vi "Dual Source Validation Utility.vi"(0 "Method File:":path=path "C:/Users/Public/Molana/Instrument/Project/MS Methods/MethodFile.xml") -> ()   [LabVIEW 2012]
uses:
  _XML Source Type.ctl
  _Source Parameter.ctl
  _Source Properties.ctl
  <vilib>/Utility/config.llb/Read Key (String).vi
  Configuration/_Global Configuration.vi
  <vilib>/xml/Close Reference(Node).vi
  <vilib>/xml/NI_XML.lvlib
  <resource>/objmgr/DOMUserDefRef.rc
  <vilib>/Utility/config.llb/NI_LVConfig.lvlib
panel:
  out "xml 2":string
  out "SourceProperties":T1[](array[typedef]) {"Source Type" items=["APCI 1", "APCI 2", "ESI 1", "ESI 2"]}
  out "Result":string="Press Load Method button to start"
  in  "Load":bool
  in  "Cancel":bool
  in  "Save As":bool
  in  "Save":bool
  out "xml":string
  in  "Current Expt":u16(ring) items=["0", "1"]
  in  "Tab":T3(tab)=enum."Experiments"
  out "Method-Level Parameter":string[][](table)
  out "Experiment List":string[][](table)
  out "Expt Comment":string
  out "Expt-Level Parameter":string[][](table)
  out "Source Type":T2 items=["APCI 1", "APCI 2", "ESI 1", "ESI 2"]
  out "Expt-Level Source Parameters":T4
  out "Mass Ranges":string[][](table)
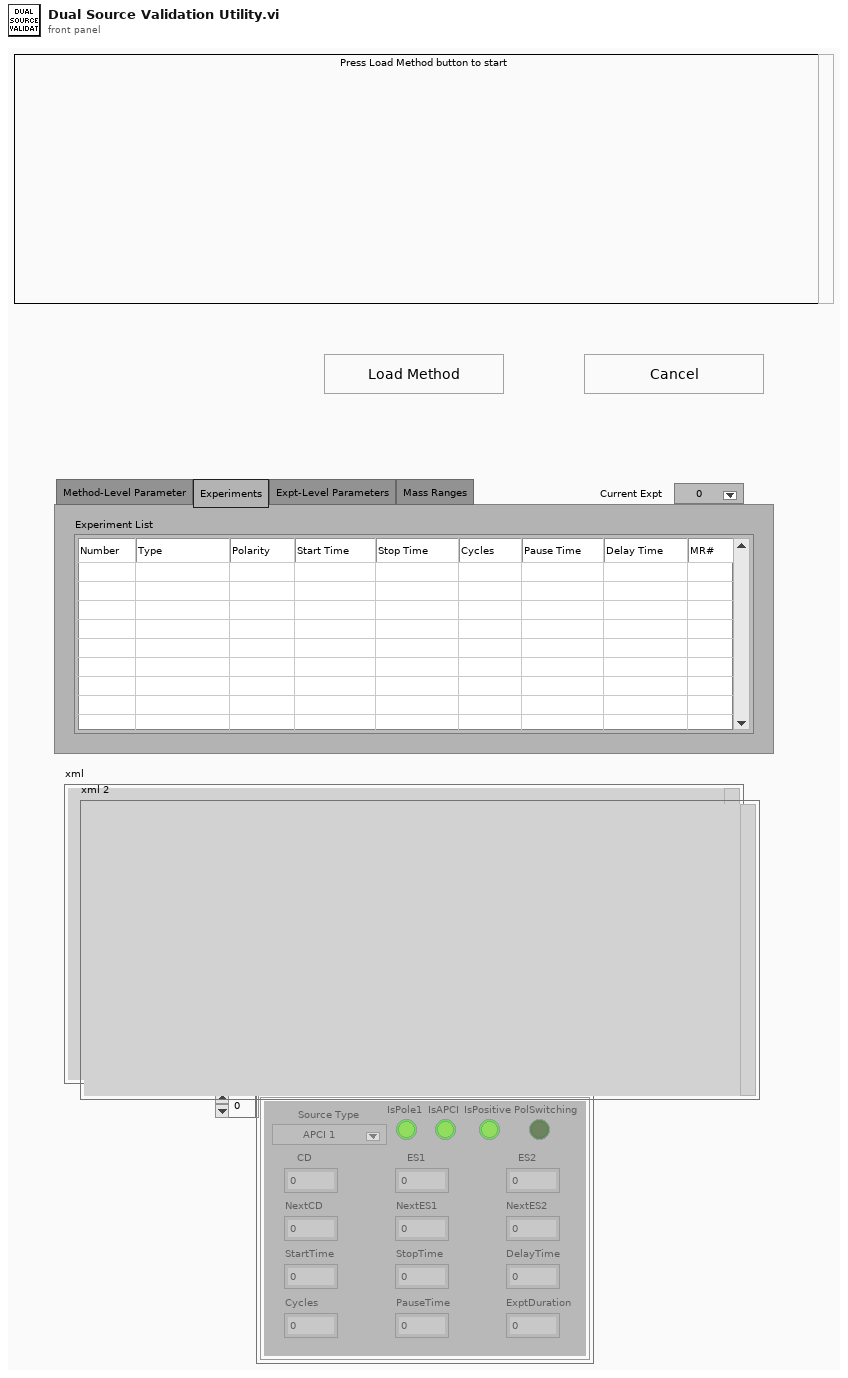
[diagram p1: front panel]
types:
  T1 = typedef "_Source Properties.ctl" = cluster{"Source Type":T2, "IsPole1":bool, "IsAPCI":bool, "IsPositive":bool, "CD":dbl, "ES1":dbl, "ES2":dbl, "NextCD":dbl, "NextES1":dbl, "NextES2":dbl, "PolSwitching":bool, "StartTime":dbl, "StopTime":dbl, "DelayTime":dbl, "Cycles":i32, "PauseTime":dbl, "ExptDuration":dbl}
  T2 = typedef "_XML Source Type.ctl" = u16
  T3 = enum32{"Method-Level Parameter", "Experiments", "Expt-Level Parameters", "Mass Ranges"}
  T4 = typedef "_Source Parameter.ctl" = cluster{"Corona Discharge: ":dbl, "ElectroSpray V1: ":dbl, "ElectroSpray V2: ":dbl}
  T5 = enum32{"existing file", "new file", "new or existing file", "existing dir", "new dir", "new or existing dir", "existing file (use LLBs)", "new file (use LLBs)", "new or existing file (use LLBs)", "new or existing file or directory (use LLBs)"}
  T6 = typedef "NI_LVConfig.lvlib/Config Data RefNum.ctl" = refnum<k1>
  T7 = typedef "_RT Instrument 2.ctl" = cluster{"Table":T8[], "Instrument":string[]}
  T8 = typedef "_RT Configuration 2.ctl" = cluster{"Name":string, "Ch#":u8, "Min":dbl, "Max":dbl, "Def+":dbl, "Def-":dbl, "Offset":dbl, "Slope":dbl, "Type":u8, "Description":string, "SettleT":dbl}
  T9 = typedef "_Mass Range Parameters.ctl" = cluster{"Name":string, "Ch#":u8, "StartV":dbl, "StopV":dbl, "StepV":dbl, "Index":u8}
  T10 = cluster{"ExptLevelParameters":string[][], "MassRanges":string[][], " MRParameters":T9[][]}
  T11 = cluster{"ExptLevelParameters":string[][], "MassRanges":string[][], " MRParameters":T9[][]}[]
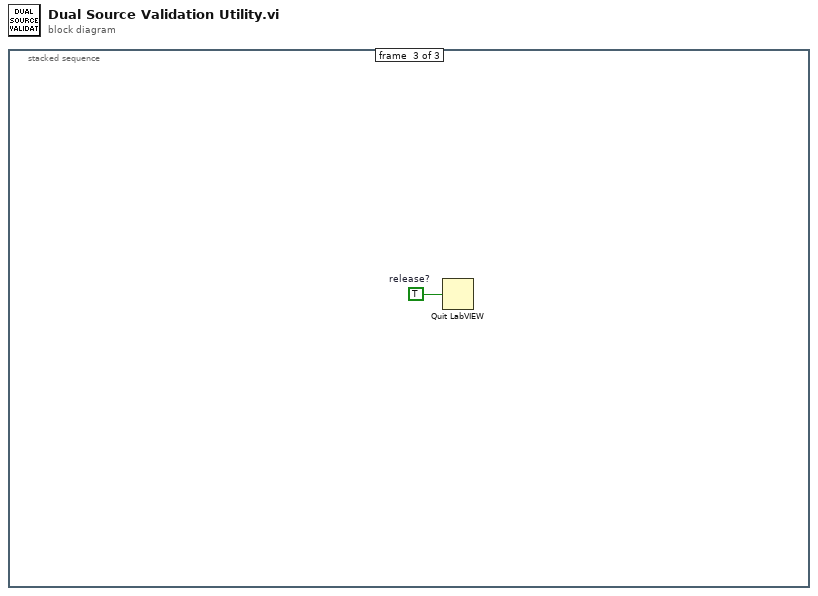
[diagram p0: block diagram]
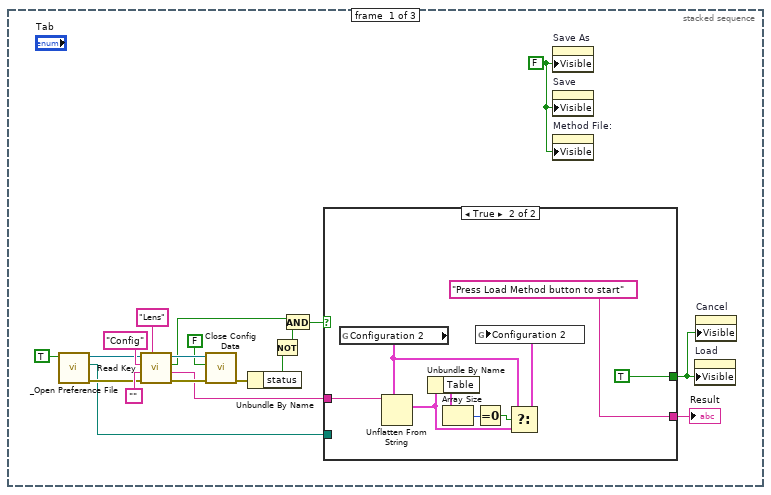
[diagram p2: hidden frame]
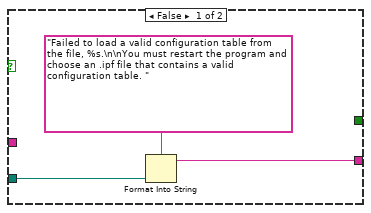
[diagram p3: hidden frame]
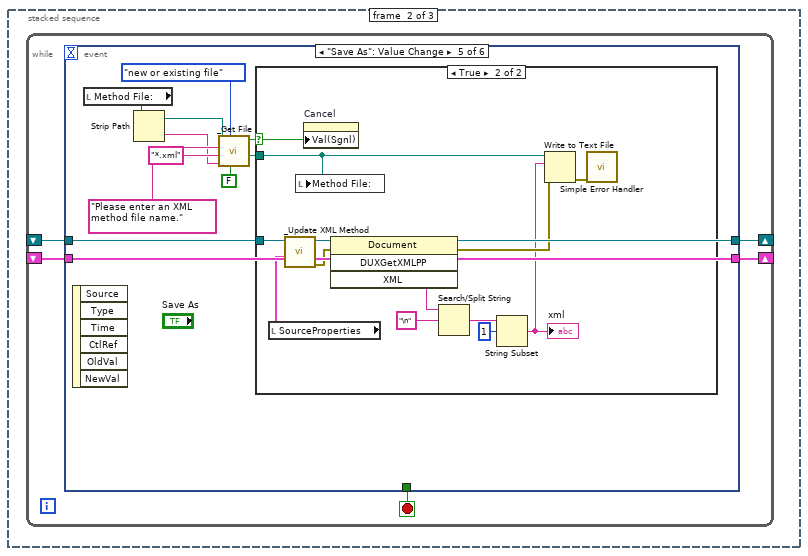
[diagram p4: hidden frame]
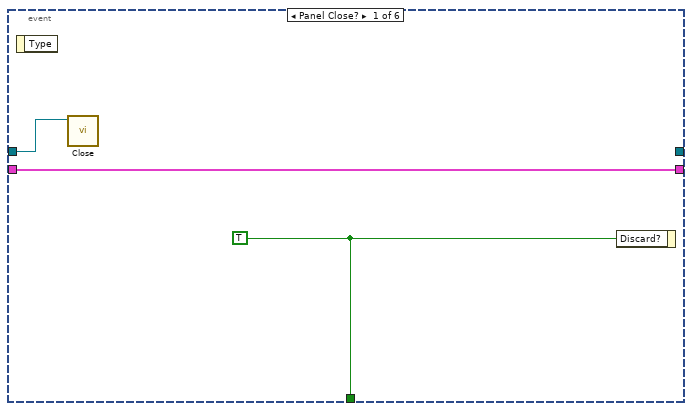
[diagram p5: hidden frame]
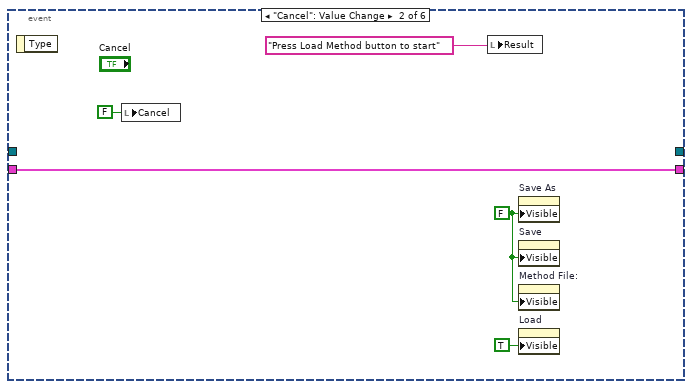
[diagram p6: hidden frame]
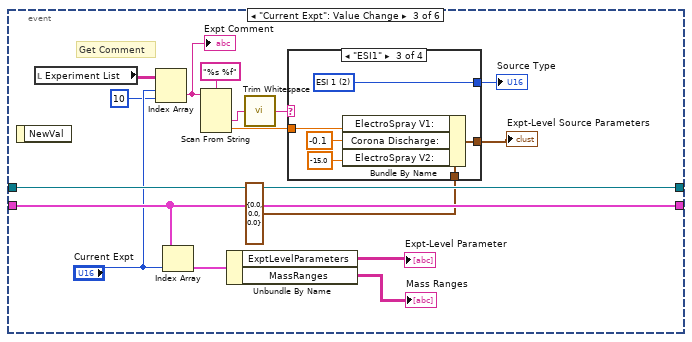
[diagram p7: hidden frame]
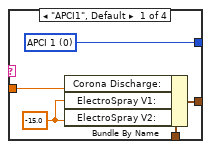
[diagram p8: hidden frame]
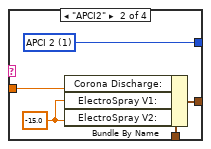
[diagram p9: hidden frame]
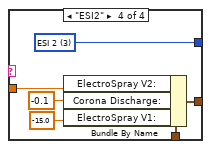
[diagram p10: hidden frame]
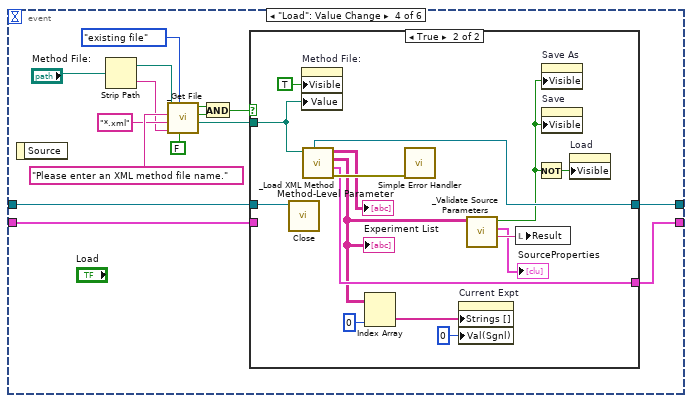
[diagram p11: hidden frame]
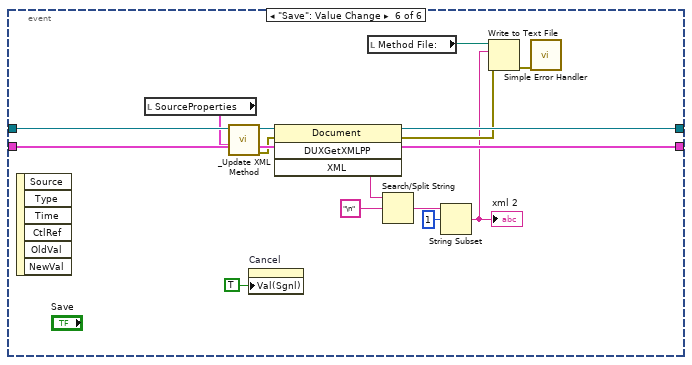
[diagram p14: hidden frame]
diagram:
  n1 = stacked-sequence {
    frame #0 {
      w7 = FALSE ("Visible")
      n2 = call "_Open Preference File.vi"("Use Designated"=TRUE) -> ("error"=w15:errorcluster, "ipf path"=w10:path, "refnum"=w16:T6)  [unwired: 4 out]
      n3 = call-poly <vilib>:"Read Key.vi"("section"="Lens", "error in (no error)"=w15, "default value"="", "key"="Config" ("section"), "refnum"=w16) -> ("error out"=w12:errorcluster, "value"=w11:string, "found?"=w3:bool, "refnum out"=w14:T6)  [unwired: 1 in, 2 out]
      n4 = call <vilib>:"Close Config Data.vi"("error in (no error)"=w12, "write file if changed (T)"=FALSE, "refnum"=w14) -> ("error out"=w6:errorcluster)  [unwired: 8 out]
      n5 = Unbundle By Name(w6) -> ("status"=w5:bool)
      n6 = Not(x=w5) -> (.not. x?=w4:bool)
      n7 = And(x=w3, y=w4) -> (x .and. y?=w2:bool)
      n8 = case shown="True" w2 {
        tunnel: w11 -> [_ w30]
        tunnel: w10 -> [w22 _]
        tunnel: [w20 "Press Load Method button to start" ("format string")] -> w8
        tunnel: [_ TRUE ("Visible")] -> w1
        frame False {
          n9 = Format Into String(format string="Failed to load a valid configuration table from the file, %s.\n\nYou must restart the program and choose an .ipf file that contains a valid configuration table. ", w22) -> (resulting string=w20:string)  [unwired: 2 in, 1 out]
        }
        frame True {
          n10 = global read "_Global Configuration.vi" "Configuration 2"() -> (w26:T7)
          n11 = Unflatten From String(type=w26, binary string=w30) -> (value=w25:T7)  [unwired: 1 in, 4 out]
          n12 = Unbundle By Name(w25) -> ("Table"=w29:T8[])
          n13 = Array Size(array=w29) -> (size(s)=w28:i32)
          n14 = Equal To 0?(x=w28) -> (x = 0?=w27:bool)
          n15 = Select(t=w26, s=w27, f=w25) -> (s? t:f=w24:T7)
          n16 = global write "_Global Configuration.vi" "Configuration 2"(w24) -> ()
        }
      }
      "Result" <- w8
      n17 = property on="Save As" class="Bool"("Visible"=w7) -> ()  [unwired: 2 in, 2 out]
      n18 = property on="Save" class="Bool"("Visible"=w7) -> ()  [unwired: 2 in, 2 out]
      n19 = property on="Method File:" class="Path"("Visible"=w7) -> ()  [unwired: 2 in, 2 out]
      n20 = property on="Load" class="Bool"("Visible"=w1) -> ()  [unwired: 2 in, 2 out]
      n21 = property on="Cancel" class="Bool (strict)"("Visible"=w1) -> ()  [unwired: 2 in, 2 out]
    }
    frame #1 {
      n22 = while {
        shift-right: [w34] -> _
        shift-left: _ -> [w35]
        shift-right: [w32] -> _
        shift-left: _ -> [w33]
        stop <- w36 stop-if-true
        n23 = event shown="[4] \"Save As\": Value Change" {
          selector: _ -> [_ _ _ _ _ _]
          dyn-events: _ -> [_ _ _ _ _ _]
          timeout: _ -> [_ _ _ _ _ _]
          tunnel: [w39 _ _ _ _ _] -> w36
          tunnel: w35 -> [w38 w44 w60 w88 w115 w151]
          tunnel: [w38 w44 w60 w89 w115 w151] -> w34
          tunnel: w33 -> [w37 _ w56 w87 w116 w152]
          tunnel: [_ _ w56 w86 w116 w152] -> w32
          event Panel Close? {
            w39 = TRUE ("Discard?")
            n24 = event-data() -> ()  [unwired: 2 out]
            n25 = call-poly <vilib>:"Close.vi"("node"=w37) -> ()  [unwired: 8 in, 1 out]
            n26 = event-data("Discard?"=w39) -> ()  [unwired: 1 in, 1 out]
          }
          event "Cancel": Value Change {
            w42 = FALSE ("Visible")
            n27 = event-data() -> ()  [unwired: 2 out]
            n28 = local write "Cancel"(FALSE ("Cancel")) -> ()
            n29 = local write "Result"("Press Load Method button to start" ("Result")) -> ()
            n30 = property on="Save As" class="Bool"("Visible"=w42) -> ()  [unwired: 2 in, 2 out]
            n31 = property on="Save" class="Bool"("Visible"=w42) -> ()  [unwired: 2 in, 2 out]
            n32 = property on="Method File:" class="Path"("Visible"=w42) -> ()  [unwired: 2 in, 2 out]
            n33 = property on="Load" class="Bool"("Visible"=TRUE) -> ()  [unwired: 2 in, 2 out]
          }
          event "Current Expt": Value Change {
            # "Get Comment"
            n34 = event-data() -> ()  [unwired: 2 out]
            n35 = local read "Experiment List"() -> (w55:string[][])
            n36 = Index Array(array=w55, index (row)="Current Expt", index (col)=10 ("disabled index (col)")) -> (element=w51:string)
            "Expt Comment" <- w51
            n37 = Index Array(array=w60, index="Current Expt") -> (element=w59:T10)
            n38 = Scan From String(format string="%s %f", input string=w51) -> (output 1=w50:string, output 2=w46:dbl)  [unwired: 4 in, 3 out]
            n39 = Unbundle By Name(w59) -> ("ExptLevelParameters"=→"Expt-Level Parameter":string[][], "MassRanges"=→"Mass Ranges":string[][])
            n40 = call <vilib>:"Trim Whitespace.vi"("string"=w50) -> ("trimmed string"=w49:string)  [unwired: 1 in]
            n41 = case shown="\"ESI1\"" w49 {
              tunnel: [w65 w70 w76 w82] -> w48
              tunnel: T4 {"Corona Discharge: "=0.0, "ElectroSpray V1: "=0.0, "ElectroSpray V2: "=0.0} ("Method-Level Source Parameters") -> [w64 w68 w73 w81]
              tunnel: w46 -> [w63 w67 w72 w80]
              tunnel: [w61 w66 w71 w77] -> w45
              frame "APCI1", Default {
                w62 = -15.0 ("ElectroSpray V2:")
                w65 = T2 0 items=["APCI 1", "APCI 2", "ESI 1", "ESI 2"] ("Source Type")
                n42 = Bundle By Name(cluster=w64, "Corona Discharge:"=w63, "ElectroSpray V1:"=w62, "ElectroSpray V2:"=w62) -> (w61:T4)
              }
              frame "APCI2" {
                w69 = -15.0 ("ElectroSpray V2:")
                w70 = T2 1 items=["APCI 1", "APCI 2", "ESI 1", "ESI 2"] ("Source Type")
                n43 = Bundle By Name(cluster=w68, "Corona Discharge:"=w67, "ElectroSpray V1:"=w69, "ElectroSpray V2:"=w69) -> (w66:T4)
              }
              frame "ESI1" {
                w76 = T2 2 items=["APCI 1", "APCI 2", "ESI 1", "ESI 2"] ("Source Type")
                n44 = Bundle By Name(cluster=w73, "ElectroSpray V1:"=w72, "Corona Discharge:"=-0.1, "ElectroSpray V2:"=-15.0) -> (w71:T4)
              }
              frame "ESI2" {
                w82 = T2 3 items=["APCI 1", "APCI 2", "ESI 1", "ESI 2"] ("Source Type")
                n45 = Bundle By Name(cluster=w81, "ElectroSpray V2:"=w80, "Corona Discharge:"=-0.1, "ElectroSpray V1:"=-15.0 ("ElectroSpray V2:")) -> (w77:T4)
              }
            }
            "Source Type" <- w48
            "Expt-Level Source Parameters" <- w45
          }
          event "Load": Value Change {
            n46 = event-data() -> ()  [unwired: 2 out]
            n47 = Strip Path(path="Method File:") -> (stripped path=w84:path, name=w83:string)
            n48 = call "_Get File.vi"("For Write (T)"=FALSE, "select mode (new or existing)"=T5."existing file", "default name"=w83, "extension (isd)"="*.xml", "prompt"="Please enter an XML method file name.", "Start Path"=w84) -> ("Seleted File"=w90:path, "Exists"=w92:bool, "Succeeded"=w93:bool)  [unwired: 1 in]
            n49 = And(x=w93, y=w92) -> (x .and. y?=w91:bool)
            n50 = case shown="True" w91 {
              tunnel: w90 -> [_ w106]
              tunnel: [w99 w112] -> w89
              tunnel: w88 -> [w99 _]
              tunnel: w87 -> [w98 w107]
              tunnel: [w98 w108] -> w86
              frame False {
              }
              frame True {
                n51 = call-poly <vilib>:"Close.vi"("node"=w107) -> ()  [unwired: 8 in, 1 out]
                n52 = property on="Method File:" class="Path"("Visible"=TRUE, "Value"=w106) -> ()  [unwired: 2 in, 2 out]
                n53 = call "_Load XML Method.vi"("Path"=w106) -> ("error out"=w114:errorcluster, "ExptParamAndMR"=w112:T11, "Experiment List"=w103:string[][], "MethodLevelParameters"=→"Method-Level Parameter":string[][], "DOM document"=w108:refnum<k20>)  [unwired: 3 in]
                "Experiment List" <- w103
                n54 = Index Array(array=w103, index (col)=0 ("disabled index (col)")) -> (element=w110:string[])  [unwired: 1 in]
                n55 = call <vilib>:"Simple Error Handler.vi"("error in (no error)"=w114) -> ()  [unwired: 4 in, 5 out]
                n56 = property on="Current Expt" class="Ring (strict)"("Strings []"=w110, "Val(Sgnl)"=u16 0 ("Value (Signaling)")) -> ()  [unwired: 2 in, 2 out]
                n57 = call "_Validate Source Parameters.vi"("Expts"=w103) -> ("Error"=w102:string, "SourceProperties"=→"SourceProperties":T1[], "Valid"=w101:bool)  [unwired: 8 in]
                n58 = local write "Result"(w102) -> ()
                n59 = Not(x=w101) -> (.not. x?=w104:bool)
                n60 = property on="Save As" class="Bool"("Visible"=w101) -> ()  [unwired: 2 in, 2 out]
                n61 = property on="Save" class="Bool"("Visible"=w101) -> ()  [unwired: 2 in, 2 out]
                n62 = property on="Load" class="Bool"("Visible"=w104) -> ()  [unwired: 2 in, 2 out]
              }
            }
          }
          event "Save As": Value Change {
            n63 = event-data() -> ()  [unwired: 7 out]
            n64 = local read "Method File:"() -> (w121:path)
            n65 = Strip Path(path=w121) -> (stripped path=w120:path, name=w119:string)
            n66 = call "_Get File.vi"("For Write (T)"=FALSE, "select mode (new or existing)"=T5."new or existing file", "default name"=w119, "extension (isd)"="*.xml", "prompt"="Please enter an XML method file name.", "Start Path"=w120) -> ("Seleted File"=w117:path, "Succeeded"=w118:bool)  [unwired: 1 in, 1 out]
            n67 = case shown="True" w118 {
              selector: w118 -> [_ w126]
              tunnel: w117 -> [_ w128]
              tunnel: w116 -> [_ w138]
              frame False {
              }
              frame True {
                n68 = local read "SourceProperties"() -> (w127:T1[])
                n69 = call "_Update XML Method.vi"("SourceProperties"=w127, "DOM document"=w138) -> ("error out"=w135:errorcluster, "DOM document out"=w137:refnum<k20>)  [unwired: 5 in]
                n70 = local write "Method File:"(w128) -> ()
                n71 = property on="Cancel" class="Bool (strict)"("Val(Sgnl)"=w126) -> ()  [unwired: 2 in, 2 out]
                n72 = invoke class="Document" method="DUXGetXMLPP"(reference=w137, error in=w135) -> (error out=w134:errorcluster, "XML"=w133:string)  [unwired: 2 in, 2 out]
                n73 = Search/Split String(string=w133, search string/char (-)="\n") -> (match + rest of string=w130:string)  [unwired: 1 in, 2 out]
                n74 = String Subset(string=w130, offset (0)=1) -> (substring=w131:string)  [unwired: 1 in]
                "xml" <- w131
                n75 = Write to Text File(file (use dialog)=w128, text=w131, error in=w134) -> (error out=w136:errorcluster)  [unwired: 1 in, 2 out]
                n76 = call <vilib>:"Simple Error Handler.vi"("error in (no error)"=w136) -> ()  [unwired: 4 in, 5 out]
              }
            }
          }
          event "Save": Value Change {
            n77 = event-data() -> ()  [unwired: 7 out]
            n78 = local read "SourceProperties"() -> (w140:T1[])
            n79 = call "_Update XML Method.vi"("SourceProperties"=w140, "DOM document"=w152) -> ("error out"=w148:errorcluster, "DOM document out"=w150:refnum<k20>)  [unwired: 5 in]
            n80 = property on="Cancel" class="Bool (strict)"("Val(Sgnl)"=TRUE ("Value (Signaling)")) -> ()  [unwired: 2 in, 2 out]
            n81 = invoke class="Document" method="DUXGetXMLPP"(reference=w150, error in=w148) -> (error out=w147:errorcluster, "XML"=w146:string)  [unwired: 2 in, 2 out]
            n82 = local read "Method File:"() -> (w141:path)
            n83 = Search/Split String(string=w146, search string/char (-)="\n") -> (match + rest of string=w143:string)  [unwired: 1 in, 2 out]
            n84 = String Subset(string=w143, offset (0)=1) -> (substring=w144:string)  [unwired: 1 in]
            "xml 2" <- w144
            n85 = Write to Text File(file (use dialog)=w141, text=w144, error in=w147) -> (error out=w149:errorcluster)  [unwired: 1 in, 2 out]
            n86 = call <vilib>:"Simple Error Handler.vi"("error in (no error)"=w149) -> ()  [unwired: 4 in, 5 out]
          }
        }
      }
    }
    frame #2 {
      w153 = TRUE  # release?
      n87 = Quit LabVIEW(quit? (T)=w153) -> ()
    }
  }
